vi "Bubble Sort.vi"(9 "Wait to View":u32=50, 11 "Unsorted Array":dbl[](array[numeric])=[7.083333333333334, 10.625, 4.791666666666667, 19.166666666666668, 10.0, 14.166666666666668, 2.916666666666667, 7.5, 18.125, 10.625, 3.125, 6.666666666666667] min=0.0 max=20.0 step=1.0) -> (2 "Partially Sorted":dbl[](array[numeric]), 3 "Sorted Array":dbl[](array[numeric]))   [LabVIEW 2015]
doc: "This VI implements bubble sort fully programmed in LabVIEW. In addition, it allows you to set a wait in the main loop and displays the partially sorted array so that you can see the actual process that bubble sort takes to sort the array"
panel:
  # "Overview: This VI implements bubble sorting of an array.\nRequirements: LabVIEW 2012 or compatible\nInstructions:\n1. Adjust the slider values in Unsorted Array to modify the values to be sorted.\n2. Set the Wait to View value to  see the actual process that bubble sort takes to sort the array in the Partially Sorted Array\n3. Run the VI"
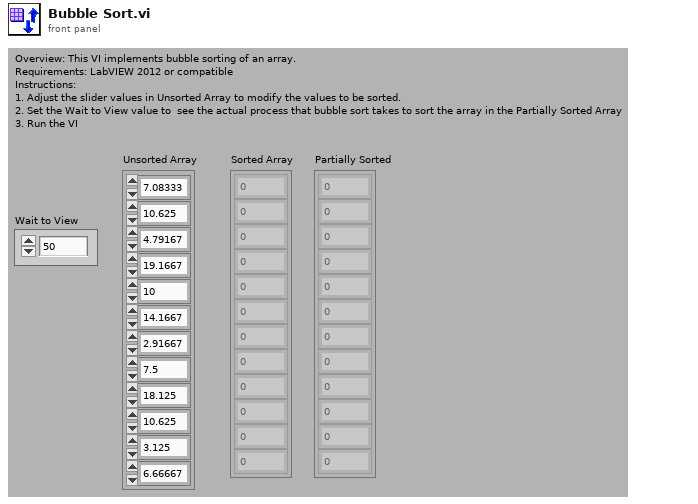
[diagram p1: front panel]
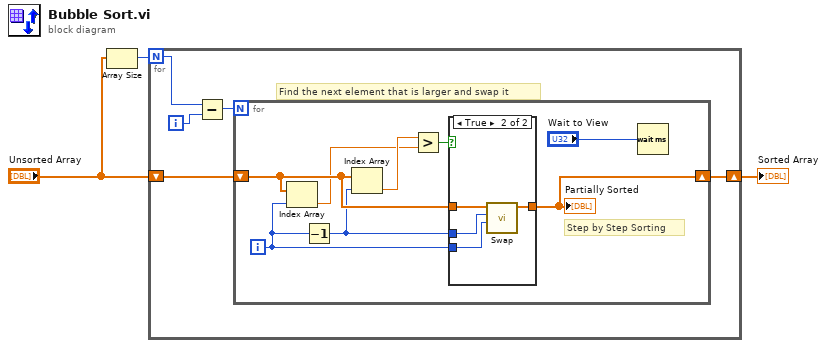
[diagram p0: block diagram]
diagram:
  n1 = Array Size(array="Unsorted Array") -> (size(s)=w3:i32)
  n2 = for {
    N: w3 -> [w7]
    shift-right: [w8] -> w1
    shift-left: "Unsorted Array" -> [w4]
    i -> [w5]
    # "Find the next element that is larger and swap it"
    n3 = Subtract(x=w7, y=w5) -> (x-y=w6:i32)
    n4 = for {
      N: w6 -> [_]
      shift-right: [w9] -> w8
      shift-left: w4 -> [w15]
      i -> [w12]
      # "Step by Step Sorting"
      n5 = Index Array(array=w15, index=w12) -> (element=w13:dbl)
      n6 = Decrement(x=w12) -> (x-1=w11:i32)
      n7 = Index Array(array=w15, index=w11) -> (element=w14:dbl)
      n8 = Greater?(x=w14, y=w13) -> (0:w16:bool)
      n9 = case shown="True" w16 {
        tunnel: w15 -> [w17 w21]
        tunnel: w11 -> [_ w20]
        tunnel: w12 -> [_ w19]
        tunnel: [w17 w18] -> w9
        frame False {
        }
        frame True {
          n10 = call "Swap.vi"("Y"=w19, "X"=w20, "Unswapped Array"=w21) -> ("Swapped Array"=w18:dbl[])  [unwired: 8 out]
        }
      }
      "Partially Sorted" <- w9
      n11 = Wait (ms)(milliseconds to wait="Wait to View") -> ()  [unwired: 1 out]
    }
  }
  "Sorted Array" <- w1
